vi "create_HDF5_file.vi"(11 "scanData":T4) -> (0 "error out":errorcluster, 1 "integration_time_dataSet":T1 {"dset_ref" format="%.0x"}, 2 "instrument_dataSet":T3 {"dset_ref" format="%.0x"}, 3 "HDF5_file_ref":T2 format="%.0x")   [LabVIEW 2015]
uses:
  controls/startScanData.ctl
  controls/scanInstrumentInfo.ctl
  <vilib>/addons/h5labview2/base/hid_t.ctl
  controls/HDF5_Dset_4d.ctl
  controls/HDF5_Dset_3d.ctl
  <vilib>/addons/h5labview2/file/H5Fmode.ctl
  <vilib>/addons/h5labview2/base/lib_path.vi
  <vilib>/addons/h5labview2/base/H5Equery.vi
  <vilib>/addons/h5labview2/attrib/H5Awrite.llb/H5Awrite.xnode
  <vilib>/addons/h5labview2/file/H5F.lvlib
  <vilib>/addons/h5labview2/dataset/H5D.lvlib
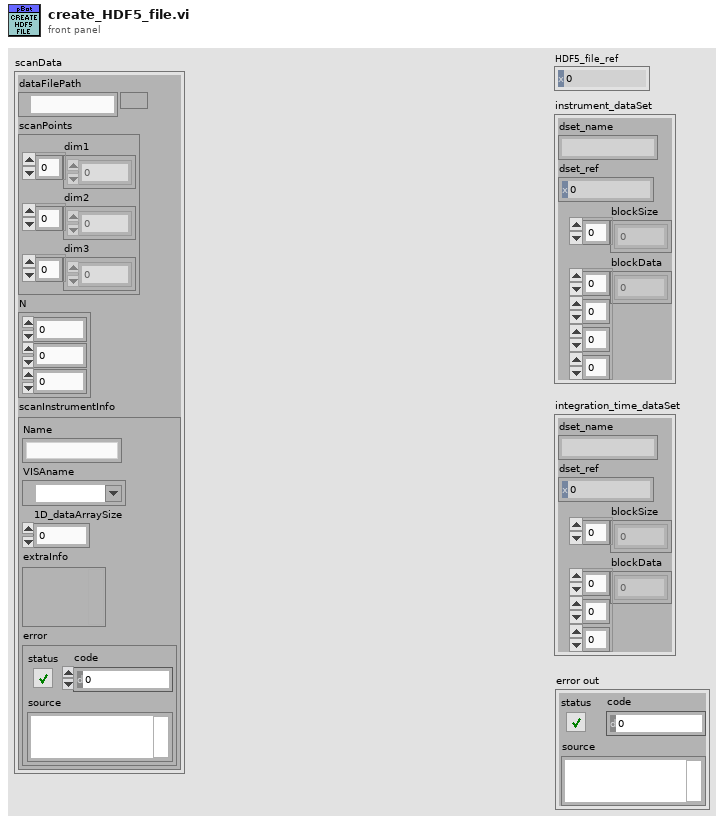
[diagram p1: front panel]
types:
  T1 = typedef "HDF5_Dset_3d.ctl" = cluster{"dset_name":string, "dset_ref":T2, "blockSize":u16[], "blockData":u32[][][]}
  T2 = typedef "hid_t.ctl" = i32
  T3 = typedef "HDF5_Dset_4d.ctl" = cluster{"dset_name":string, "dset_ref":T2, "blockSize":u16[], "blockData":u16[][][][]}
  T4 = typedef "startScanData.ctl" = cluster{"dataFilePath":path, "scanPoints":cluster{"dim1":sgl[], "dim2":sgl[], "dim3":sgl[]}, "N":cluster{"X":u16, "Y":u16, "Z":u16}, "scanInstrumentInfo":T5}
  T5 = typedef "scanInstrumentInfo.ctl" = cluster{"Name":string, "VISAname":refnum<visa-resource-name>, "1D_dataArraySize":u16, "extraInfo":variant, "error":errorcluster}
  T6 = typedef "H5F.lvlib/H5Fmode.ctl" = enum16{"read-only", "read-write", "overwrite", "create new", "open or create"}
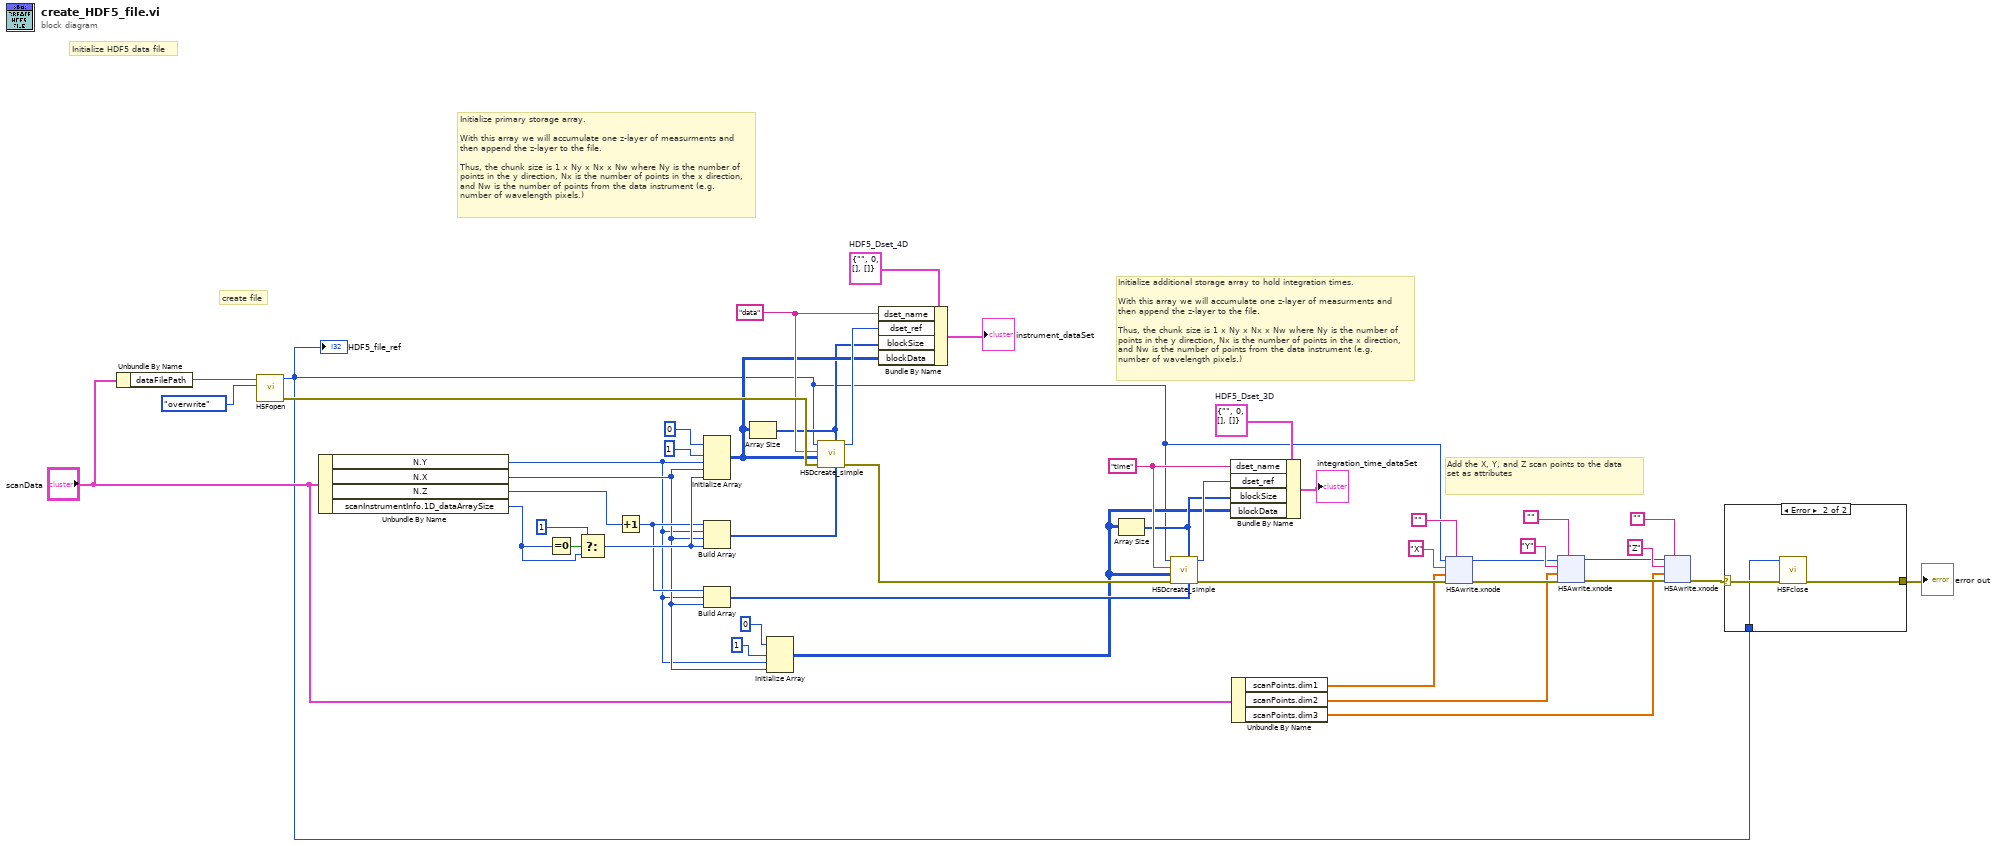
[diagram p0: block diagram]
diagram:
  w10 = T1 {"dset_name"="", "dset_ref"=0, "blockSize"=[], "blockData"=[]}  # HDF5_Dset_3D
  w15 = T3 {"dset_name"="", "dset_ref"=0, "blockSize"=[], "blockData"=[]}  # HDF5_Dset_4D
  w9 = "time" ("name")
  w14 = "data" ("name")
  # "Add the X, Y, and Z scan points to the data set as attributes"
  # "Initialize additional storage array to hold integration times.\n\nWith this array we will accumulate one z-layer of measurments and then append the z-layer to the file.\n\nThus, the chunk size is 1 x Ny x Nx x Nw where Ny is the number of points in the y direction, Nx is the number of points in the x direction, and Nw is the number of points from the data instrument (e.g. number of wavelength pixels.)"
  # "Initialize primary storage array.\n\nWith this array we will accumulate one z-layer of measurments and then append the z-layer to the file.\n\nThus, the chunk size is 1 x Ny x Nx x Nw where Ny is the number of points in the y direction, Nx is the number of points in the x direction, and Nw is the number of points from the data instrument (e.g. number of wavelength pixels.)"
  # "create file"
  # "Initialize HDF5 data file"
  n1 = Unbundle By Name("scanData") -> ("dataFilePath"=w38:path)
  n2 = call <vilib>:"H5Fopen.vi"("mode (read-only)"=H5Fmode."overwrite" ("mode"), "path"=w38) -> ("error out"=w39:errorcluster, "ref out"=w1:T2)  [unwired: 8 in]
  "HDF5_file_ref" <- w1
  n3 = Unbundle By Name("scanData") -> ("N.Y"=w31:u16, "N.X"=w32:u16, "N.Z"=w41:u16, "scanInstrumentInfo.1D_dataArraySize"=w46:u16)
  n4 = Equal To 0?(x=w46) -> (x = 0?=w47:bool)
  n5 = Select(t=u16 1, s=w47, f=w46) -> (s? t:f=w42:u16)
  n6 = Increment(x=w41) -> (x+1=w36:u16)
  n7 = Initialize Array(u16 0 ("element"), u32 1 ("dimension size"), w31, w32, w42) -> (w12:u16[][][][])
  n8 = Build Array(w36, w31, w32, w42) -> (w40:u16[])
  n9 = Build Array(w36, w31, w32) -> (w35:u16[])
  n10 = Array Size(array=w12) -> (size(s)=w11:i32[])
  n11 = Initialize Array(u32 0 ("element"), u32 1 ("dimension size"), w31, w32) -> (w6:u32[][][])
  n12 = call <vilib>:"H5Dcreate_simple.vi"("max size"=w40, "chunk size"=w11, "error in (no error)"=w39, "type in"=w12, "name"=w14, "ref in"=w1) -> ("error out"=w37:errorcluster, "dset out"=w13:T2)  [unwired: 4 in]
  n13 = Bundle By Name(cluster=w15, "dset_name"=w14, "dset_ref"=w13, "blockSize"=w11, "blockData"=w12) -> (→"instrument_dataSet":T3)
  n14 = Array Size(array=w6) -> (size(s)=w7:i32[])
  n15 = call <vilib>:"H5Dcreate_simple.vi"("max size"=w35, "chunk size"=w7, "error in (no error)"=w37, "type in"=w6, "name"=w9, "ref in"=w1) -> ("error out"=w28:errorcluster, "dset out"=w8:T2)  [unwired: 4 in]
  n16 = Bundle By Name(cluster=w10, "dset_name"=w9, "dset_ref"=w8, "blockSize"=w7, "blockData"=w6) -> (→"integration_time_dataSet":T1)
  n17 = Unbundle By Name("scanData") -> ("scanPoints.dim1"=w18:sgl[], "scanPoints.dim2"=w17:sgl[], "scanPoints.dim3"=w16:sgl[])
  n18 = xnode "H5Awrite.xnode"("object name"="", "error in (no error)"=w28, "data"=w18, "attrib name"="X", "ref in"=w1) -> ("error out"=w21:errorcluster, "ref out"=w23:T2)  [unwired: 2 in, 1 out]
  n19 = xnode "H5Awrite.xnode"("object name"="", "error in (no error)"=w21, "data"=w17, "attrib name"="Y", "ref in"=w23) -> ("error out"=w20:errorcluster, "ref out"=w22:T2)  [unwired: 2 in, 1 out]
  n20 = xnode "H5Awrite.xnode"("object name"="", "error in (no error)"=w20, "data"=w16, "attrib name"="Z", "ref in"=w22) -> ("error out"=w5:errorcluster)  [unwired: 2 in, 2 out]
  n21 = case shown="Error" w5 {
    selector: w5 -> [w49 w52]
    tunnel: w1 -> [_ w51]
    tunnel: [w49 w50] -> w4
    frame No Error {
    }
    frame Error {
      n22 = call <vilib>:"H5Fclose.vi"("error in (no error)"=w52, "ref"=w51) -> ("error out"=w50:errorcluster)  [unwired: 9 in]
    }
  }
  "error out" <- w4
